vi "Cluster to Array of Variants.vi"(11 "Cluster":variant) -> (2 "Names":string[](array[string]), 3 "Data":variant[](array[variant]))   [LabVIEW 2020, in "Advanced Assertions.lvlib"]
uses:
  Advanced Assertions.lvlib
panel:
  out "xml string":string
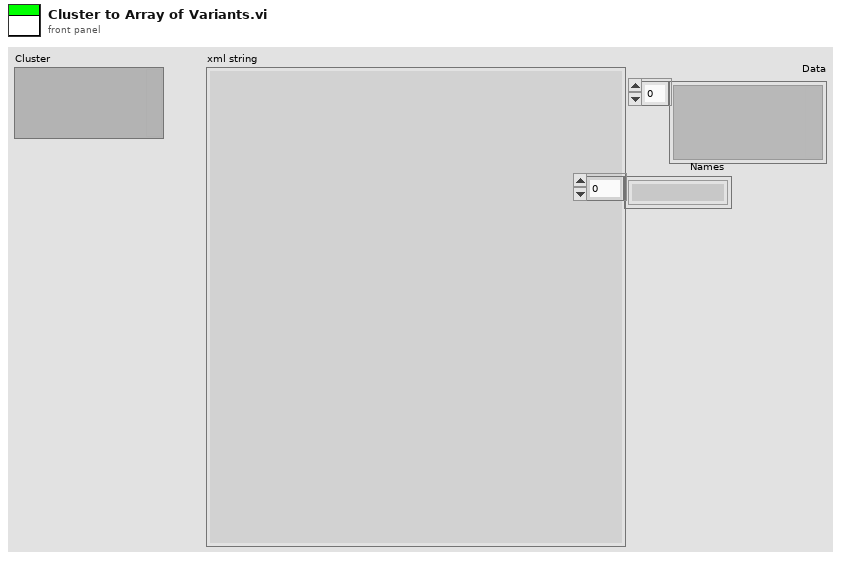
[diagram p1: front panel]
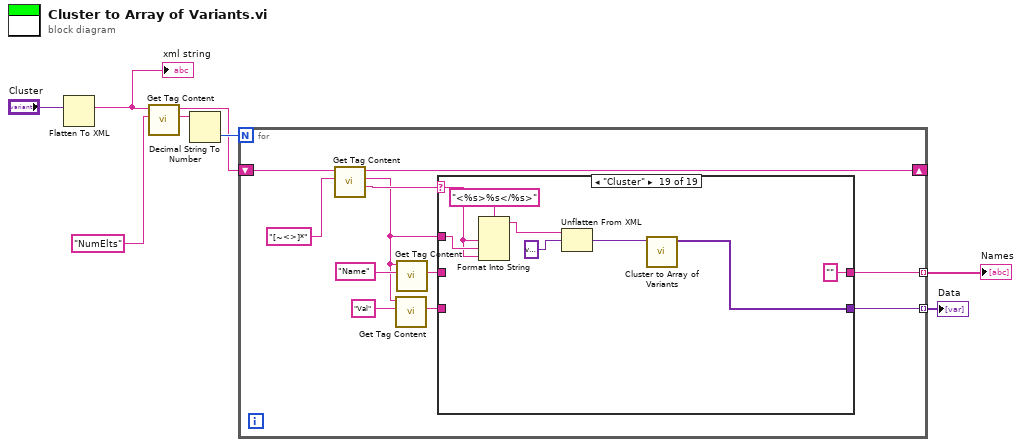
[diagram p0: block diagram]
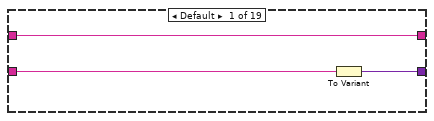
[diagram p2: hidden frame]
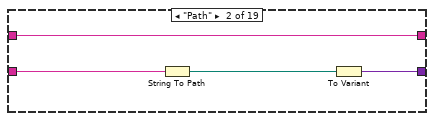
[diagram p3: hidden frame]
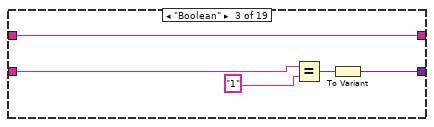
[diagram p4: hidden frame]
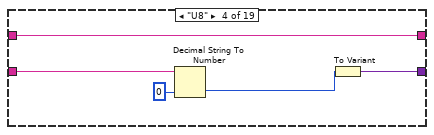
[diagram p5: hidden frame]
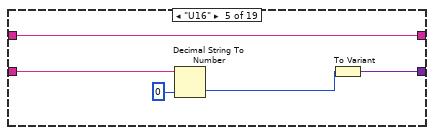
[diagram p6: hidden frame]
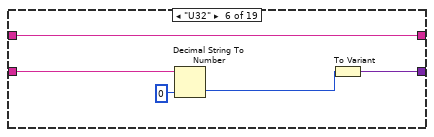
[diagram p7: hidden frame]
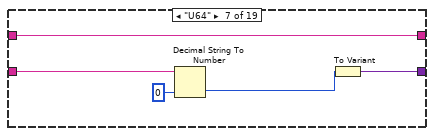
[diagram p8: hidden frame]
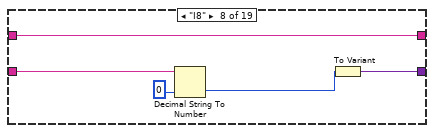
[diagram p9: hidden frame]
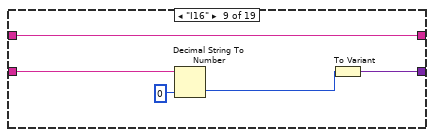
[diagram p10: hidden frame]
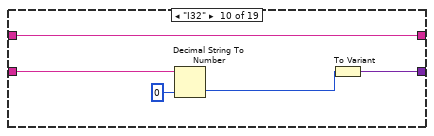
[diagram p11: hidden frame]
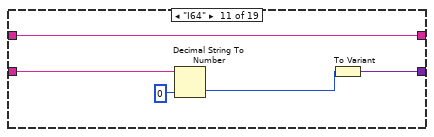
[diagram p12: hidden frame]
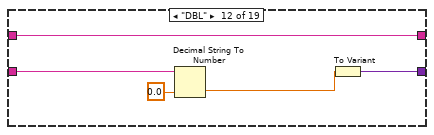
[diagram p13: hidden frame]
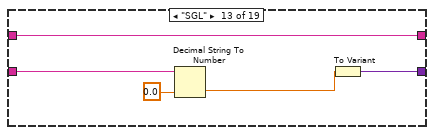
[diagram p14: hidden frame]
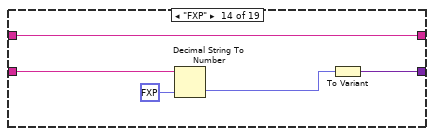
[diagram p15: hidden frame]
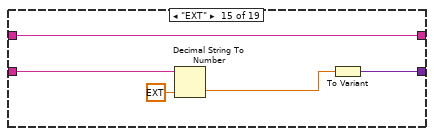
[diagram p16: hidden frame]
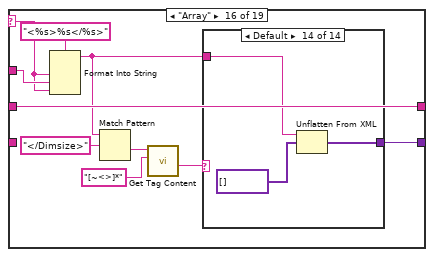
[diagram p17: hidden frame]
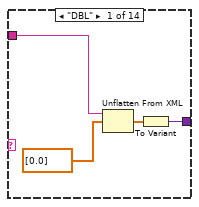
[diagram p18: hidden frame]
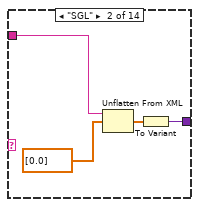
[diagram p19: hidden frame]
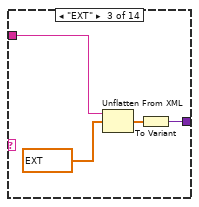
[diagram p20: hidden frame]
diagram:
  n1 = Flatten To XML(6:"Cluster") -> (2:w2:string)
  "xml string" <- w2
  n2 = call "Get Tag Content.vi"("Tag"="NumElts" ("regular expression"), "xml string in"=w2) -> ("Tag content"=w3:string, "After end of tag"=w1:string)  [unwired: 7 in, 1 out]
  n3 = Decimal String To Number(string=w3) -> (number=w4:i32)  [unwired: 2 in, 1 out]
  n4 = for {
    N: w4 -> [_]
    tunnel: [w15] -> w5 mode=indexing
    tunnel: [w16] -> w6 mode=indexing
    shift-right: [w17] -> _
    shift-left: w1 -> [w19]
    n5 = call "Get Tag Content.vi"("Tag"="[~<>]*" ("regular expression"), "xml string in"=w19) -> ("Type"=w14:string, "Tag content"=w9:string, "After end of tag"=w17:string)  [unwired: 7 in]
    n6 = call "Get Tag Content.vi"("Tag"="Val" ("regular expression"), "xml string in"=w9) -> ("Tag content"=w10:string)  [unwired: 7 in, 2 out]
    n7 = call "Get Tag Content.vi"("Tag"="Name" ("regular expression"), "xml string in"=w9) -> ("Tag content"=w11:string)  [unwired: 7 in, 2 out]
    n8 = case shown="\"Cluster\"" w14 {
      selector: w14 -> [_ _ _ _ _ _ _ _ _ _ _ _ _ _ _ w97 w160 w168 w177]
      tunnel: [w21 w25 w28 w35 w40 w45 w50 w55 w60 w65 w70 w75 w80 w85 w90 w101 w164 w171 "" ("Tag content")] -> w16
      tunnel: [w22 w26 w29 w36 w41 w46 w51 w56 w61 w66 w71 w76 w81 w86 w91 w100 w163 w165 w173] -> w15
      tunnel: w11 -> [w21 w25 w28 w35 w40 w45 w50 w55 w60 w65 w70 w75 w80 w85 w90 w101 w164 w171 _]
      tunnel: w10 -> [w20 w24 w27 w34 w39 w44 w49 w54 w59 w64 w69 w74 w79 w84 w89 _ _ _ _]
      tunnel: w9 -> [_ _ _ _ _ _ _ _ _ _ _ _ _ _ _ w99 w162 w170 w179]
      frame Default {
        n9 = To Variant(anything=w20) -> (Variant=w22:variant)
      }
      frame "Path" {
        n10 = String To Path(string=w24) -> (path=w23:path)
        n11 = To Variant(anything=w23) -> (Variant=w26:variant)
      }
      frame "Boolean" {
        n12 = Equal?(x=w27, y="1") -> (x = y?=w31:bool)
        n13 = To Variant(anything=w31) -> (Variant=w29:variant)
      }
      frame "U8" {
        n14 = Decimal String To Number(string=w34, default (0L)=u8 0 ("default (0 I32)")) -> (number=w33:u8)  [unwired: 1 in, 1 out]
        n15 = To Variant(anything=w33) -> (Variant=w36:variant)
      }
      frame "U16" {
        n16 = Decimal String To Number(string=w39, default (0L)=u16 0 ("default (0 I32)")) -> (number=w38:u16)  [unwired: 1 in, 1 out]
        n17 = To Variant(anything=w38) -> (Variant=w41:variant)
      }
      frame "U32" {
        n18 = Decimal String To Number(string=w44, default (0L)=u32 0 ("default (0 I32)")) -> (number=w43:u32)  [unwired: 1 in, 1 out]
        n19 = To Variant(anything=w43) -> (Variant=w46:variant)
      }
      frame "U64" {
        n20 = Decimal String To Number(string=w49, default (0L)=u64 0 ("default (0 I32)")) -> (number=w48:u64)  [unwired: 1 in, 1 out]
        n21 = To Variant(anything=w48) -> (Variant=w51:variant)
      }
      frame "I8" {
        n22 = Decimal String To Number(string=w54, default (0L)=i8 0 ("default (0 I32)")) -> (number=w53:i8)  [unwired: 1 in, 1 out]
        n23 = To Variant(anything=w53) -> (Variant=w56:variant)
      }
      frame "I16" {
        n24 = Decimal String To Number(string=w59, default (0L)=i16 0 ("default (0 I32)")) -> (number=w58:i16)  [unwired: 1 in, 1 out]
        n25 = To Variant(anything=w58) -> (Variant=w61:variant)
      }
      frame "I32" {
        n26 = Decimal String To Number(string=w64, default (0L)=0 ("default (0 I32)")) -> (number=w63:i32)  [unwired: 1 in, 1 out]
        n27 = To Variant(anything=w63) -> (Variant=w66:variant)
      }
      frame "I64" {
        n28 = Decimal String To Number(string=w69, default (0L)=i64 0 ("default (0 I32)")) -> (number=w68:i64)  [unwired: 1 in, 1 out]
        n29 = To Variant(anything=w68) -> (Variant=w71:variant)
      }
      frame "DBL" {
        n30 = Decimal String To Number(string=w74, default (0L)=0.0 ("default (0 I32)")) -> (number=w73:dbl)  [unwired: 1 in, 1 out]
        n31 = To Variant(anything=w73) -> (Variant=w76:variant)
      }
      frame "SGL" {
        n32 = Decimal String To Number(string=w79, default (0L)=sgl 0.0 ("default (0 I32)")) -> (number=w78:sgl)  [unwired: 1 in, 1 out]
        n33 = To Variant(anything=w78) -> (Variant=w81:variant)
      }
      frame "FXP" {
        n34 = Decimal String To Number(string=w84, default (0L)=fxp<+,1,1> 0.0 ("default (0 I32)")) -> (number=w82:fxp<+,1,1>)  [unwired: 1 in, 1 out]
        n35 = To Variant(anything=w82) -> (Variant=w86:variant)
      }
      frame "EXT" {
        n36 = Decimal String To Number(string=w89, default (0L)=ext 0.0 ("default (0 I32)")) -> (number=w87:ext)  [unwired: 1 in, 1 out]
        n37 = To Variant(anything=w87) -> (Variant=w91:variant)
      }
      frame "Array" {
        n38 = Format Into String(format string="<%s>%s</%s>", w97, w99, w97) -> (resulting string=w96:string)  [unwired: 2 in, 1 out]
        n39 = Match Pattern(string=w96, regular expression="</Dimsize>") -> (after substring=w94:string)  [unwired: 1 in, 3 out]
        n40 = call "Get Tag Content.vi"("Tag"="[~<>]*" ("regular expression"), "xml string in"=w94) -> ("Type"=w92:string)  [unwired: 7 in, 2 out]
        n41 = case shown="Default" w92 {
          tunnel: [w103 w107 w111 w115 w119 w123 w127 w131 w135 w139 w143 w147 w151 w154] -> w100
          tunnel: w96 -> [w102 w106 w110 w114 w118 w122 w126 w130 w134 w138 w142 w146 w150 w155]
          frame "DBL" {
            n42 = Unflatten From XML(xml string=w102, type=dbl[] [0.0]) -> (value=w104:dbl[])  [unwired: 1 in, 1 out]
            n43 = To Variant(anything=w104) -> (Variant=w103:variant)
          }
          frame "SGL" {
            n44 = Unflatten From XML(xml string=w106, type=sgl[] [0.0]) -> (value=w108:sgl[])  [unwired: 1 in, 1 out]
            n45 = To Variant(anything=w108) -> (Variant=w107:variant)
          }
          frame "EXT" {
            n46 = Unflatten From XML(xml string=w110, type=ext[] [0.0]) -> (value=w112:ext[])  [unwired: 1 in, 1 out]
            n47 = To Variant(anything=w112) -> (Variant=w111:variant)
          }
          frame "FXP" {
            n48 = Unflatten From XML(xml string=w114, type=fxp<+,1,1>[] [0.0]) -> (value=w116:fxp<+,1,1>[])  [unwired: 1 in, 1 out]
            n49 = To Variant(anything=w116) -> (Variant=w115:variant)
          }
          frame "I64" {
            n50 = Unflatten From XML(xml string=w118, type=i64[] [0]) -> (value=w120:i64[])  [unwired: 1 in, 1 out]
            n51 = To Variant(anything=w120) -> (Variant=w119:variant)
          }
          frame "I32" {
            n52 = Unflatten From XML(xml string=w122, type=i32[] [0]) -> (value=w124:i32[])  [unwired: 1 in, 1 out]
            n53 = To Variant(anything=w124) -> (Variant=w123:variant)
          }
          frame "I16" {
            n54 = Unflatten From XML(xml string=w126, type=i16[] [0]) -> (value=w128:i16[])  [unwired: 1 in, 1 out]
            n55 = To Variant(anything=w128) -> (Variant=w127:variant)
          }
          frame "I8" {
            n56 = Unflatten From XML(xml string=w130, type=i8[] [0]) -> (value=w132:i8[])  [unwired: 1 in, 1 out]
            n57 = To Variant(anything=w132) -> (Variant=w131:variant)
          }
          frame "U64" {
            n58 = Unflatten From XML(xml string=w134, type=u64[] [0]) -> (value=w136:u64[])  [unwired: 1 in, 1 out]
            n59 = To Variant(anything=w136) -> (Variant=w135:variant)
          }
          frame "U32" {
            n60 = Unflatten From XML(xml string=w138, type=u32[] [0]) -> (value=w140:u32[])  [unwired: 1 in, 1 out]
            n61 = To Variant(anything=w140) -> (Variant=w139:variant)
          }
          frame "U16" {
            n62 = Unflatten From XML(xml string=w142, type=u16[] [0]) -> (value=w144:u16[])  [unwired: 1 in, 1 out]
            n63 = To Variant(anything=w144) -> (Variant=w143:variant)
          }
          frame "U8" {
            n64 = Unflatten From XML(xml string=w146, type=u8[] [0]) -> (value=w148:u8[])  [unwired: 1 in, 1 out]
            n65 = To Variant(anything=w148) -> (Variant=w147:variant)
          }
          frame "String" {
            n66 = Unflatten From XML(xml string=w150, type=string[] [""]) -> (value=w152:string[])  [unwired: 1 in, 1 out]
            n67 = To Variant(anything=w152) -> (Variant=w151:variant)
          }
          frame Default {
            n68 = Unflatten From XML(xml string=w155, type=variant[] []) -> (value=w154:variant[])  [unwired: 1 in, 1 out]
          }
        }
      }
      frame "Timestamp" {
        n69 = Format Into String(format string="<%s>%s</%s>", w160, w162, w160) -> (resulting string=w159:string)  [unwired: 2 in, 1 out]
        n70 = Unflatten From XML(xml string=w159, type=timestamp(0 s since 1904-01-01)) -> (value=w158:timestamp)  [unwired: 1 in, 1 out]
        n71 = To Variant(anything=w158) -> (Variant=w163:variant)
      }
      frame "EB", "EL", "EW" {
        n72 = Format Into String(format string="<%s>%s</%s>", w168, w170, w168) -> (resulting string=w167:string)  [unwired: 2 in, 1 out]
        n73 = Unflatten From XML(xml string=w167, type=variant) -> (value=w165:variant)  [unwired: 1 in, 1 out]
      }
      frame "Cluster" {
        n74 = Format Into String(format string="<%s>%s</%s>", w177, w179, w177) -> (resulting string=w176:string)  [unwired: 2 in, 1 out]
        n75 = Unflatten From XML(xml string=w176, type=variant) -> (value=w174:variant)  [unwired: 1 in, 1 out]
        n76 = call "Cluster to Array of Variants.vi"("Cluster"=w174) -> ("Data"=w173:variant[])  [unwired: 9 in, 1 out]
      }
    }
  }
  "Data" <- w5
  "Names" <- w6
